vi "Indices (1D) to One-Hot (3D).vi"(1 "# Embedding Dimensions":i32=5, 4 "indices":i64[](array[numeric])=[0, 1, 4]) -> (15 "Array of One-Hots":dbl[][][](array[numeric])=[[[1.0], [0.0], [0.0], [0.0], [0.0]], [[0.0], [1.0], [0.0], [0.0], [0.0]], [[0.0], [0.0], [0.0], [0.0], [1.0]]])   [LabVIEW 2014]
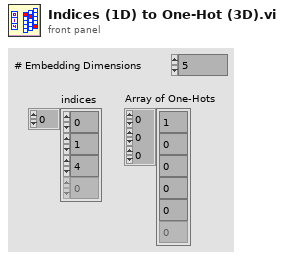
[diagram p1: front panel]
types:
  T1 = typedef "NI_Matrix.lvlib/RealMatrix.ctl" = dbl[][]
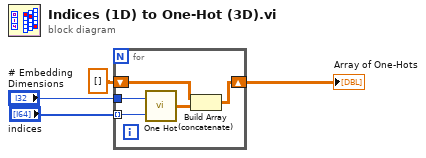
[diagram p0: block diagram]
diagram:
  n1 = for {
    shift-right: [w7] -> w4
    shift-left: dbl[][][] [] -> [w5]
    tunnel: "indices" -> [w9] mode=indexing
    tunnel: "# Embedding Dimensions" -> [w8]
    n2 = call "One Hot.vi"("hot index"=w9, "length"=w8) -> ("One hot vector"=w6:T1)
    n3 = Build Array (concatenate)(w5, w6) -> (w7:dbl[][][])
  }
  "Array of One-Hots" <- w4
